vi "cut_gps_speed_data.vi"(8 "gps shift [s]":dbl format="%#_13g", 9 "Sec":dbl format="%#_13g", 10 "Start Time":timestamp, 11 "timestamp gps speed data":cluster{timestamp[], dbl[]}) -> (3 "XY gps speed data":cluster{dbl[], dbl[]})   [LabVIEW 2020]
panel:
  out "out":cluster{dbl[], dbl[]}(graph)
  out "in":cluster{timestamp[], dbl[]}(graph)
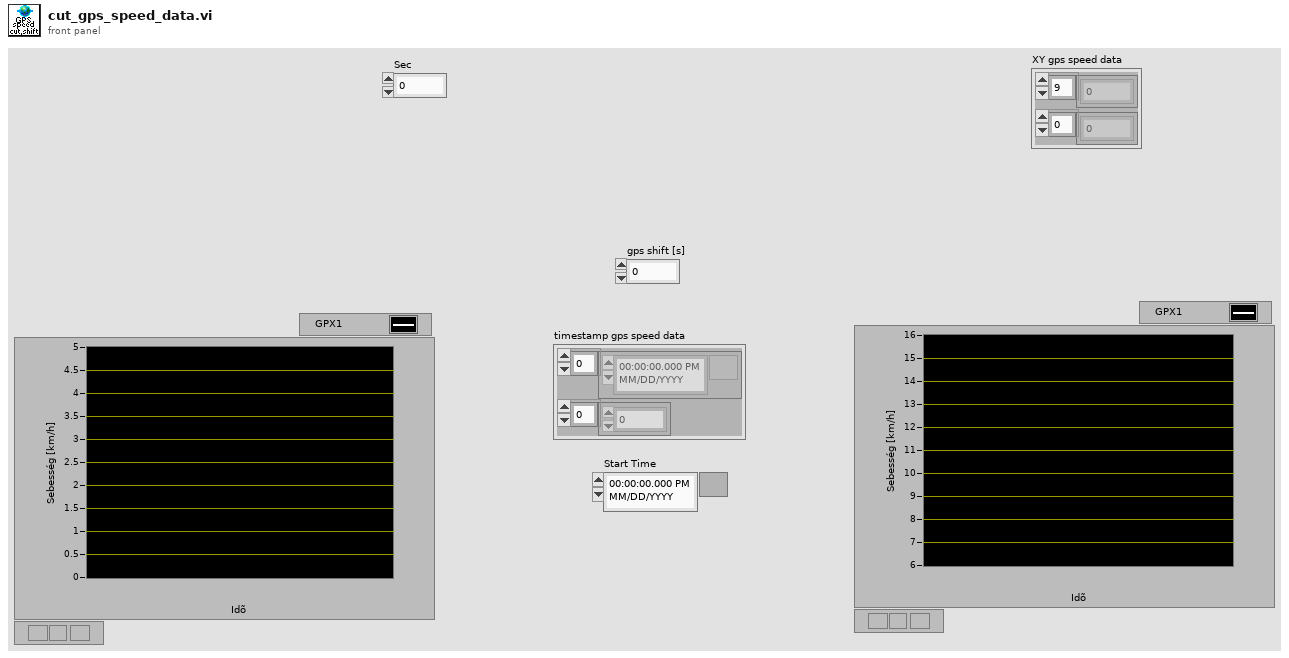
[diagram p1: front panel]
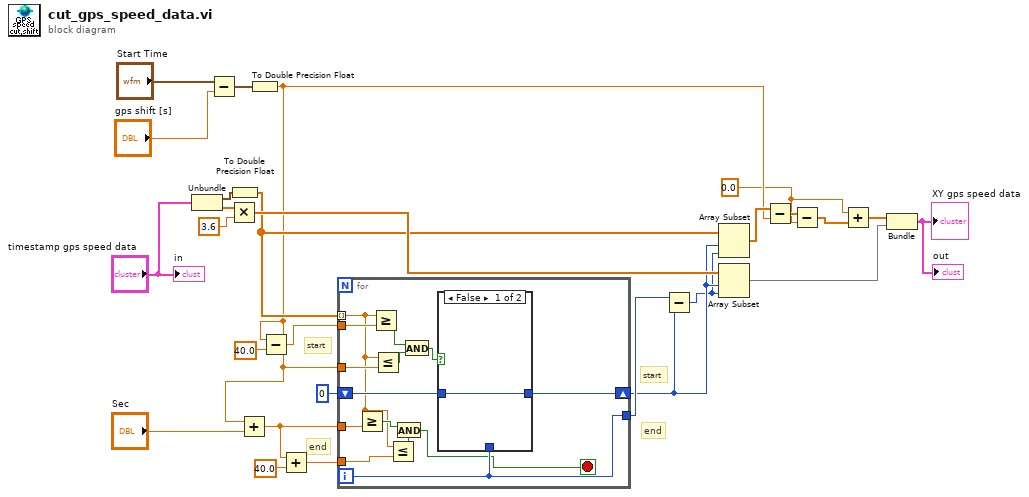
[diagram p0: block diagram]
diagram:
  w1 = 0.0 ("x")
  # "end"
  # "start"
  # "end"
  # "start"
  n1 = Unbundle("timestamp gps speed data") -> (w25:timestamp[], w27:dbl[])
  n2 = Subtract(x="Start Time", y="gps shift [s]") -> (x-y=w12:timestamp)
  n3 = Multiply(x=w27, y=3.6) -> (x*y=w19:dbl[])
  n4 = To Double Precision Float(number=w25) -> (double precision float=w14:dbl[])
  n5 = To Double Precision Float(number=w12) -> (double precision float=w3:dbl)
  n6 = Add(x=w3, y="Sec") -> (x+y=w2:dbl)
  n7 = Subtract(x=w3, y=40.0) -> (x-y=w22:dbl)
  n8 = Add(x=w2, y=40.0) -> (x+y=w20:dbl)
  n9 = for {
    tunnel: w22 -> [w35]
    tunnel: w14 -> [w28] mode=indexing
    shift-right: [w41] -> w16
    shift-left: 0 -> [w40]
    tunnel: w2 -> [w34]
    tunnel: [w39] -> w17
    tunnel: w3 -> [w30]
    tunnel: w20 -> [w29]
    i -> [w39]
    stop <- w31 stop-if-true
    n10 = Greater Or Equal?(x=w28, y=w34) -> (x >= y?=w33:bool)
    n11 = Greater Or Equal?(x=w28, y=w35) -> (x >= y?=w37:bool)
    n12 = Less Or Equal?(x=w28, y=w30) -> (x <= y?=w36:bool)
    n13 = Less Or Equal?(x=w28, y=w29) -> (x <= y?=w32:bool)
    n14 = And(x=w33, y=w32) -> (x .and. y?=w31:bool)
    n15 = And(x=w37, y=w36) -> (x .and. y?=w38:bool)
    n16 = case shown="False" w38 {
      tunnel: [w42 w43] -> w41
      tunnel: w39 -> [_ w43]
      tunnel: w40 -> [w42 _]
      frame False {
      }
      frame True {
      }
    }
  }
  n17 = Subtract(x=w17, y=w16) -> (x-y=w15:i32)
  n18 = Array Subset(array=w14, index=w16, length=w15) -> (w13:dbl[])
  n19 = Array Subset(array=w19, index=w16, length=w15) -> (w18:dbl[])
  n20 = Subtract(x=w13, y=w3) -> (x-y=w7:dbl[])
  n21 = Subtract(x=w7, y=w1) -> (x-y=w5:dbl[])
  n22 = Add(x=w1, y=w5) -> (x+y=w6:dbl[])
  n23 = Bundle(w6, w18) -> (→"XY gps speed data" →"out":cluster{dbl[], dbl[]})  [unwired: 1 in]
  "in" <- "timestamp gps speed data"
